vi "Get Camera Configuration.vi"(8 "error in (no error)":errorcluster, 11 "NI Vision Camera Device in":refnum<class "NI Vision Camera Device.lvclass">) -> (0 "error out":errorcluster, 2 "Configuration":T1, 3 "NI Vision Camera Device out":refnum<class "NI Vision Camera Device.lvclass">)   [LabVIEW 2014, in "NI Vision Camera Device.lvclass"]
uses:
  NI Vision Camera Device.lvclass
  Configuration.ctl
  NI Vision Camera Device.lvclass/NI Vision Camera Device.ctl
  <resource>/objmgr/imaqdx.rc
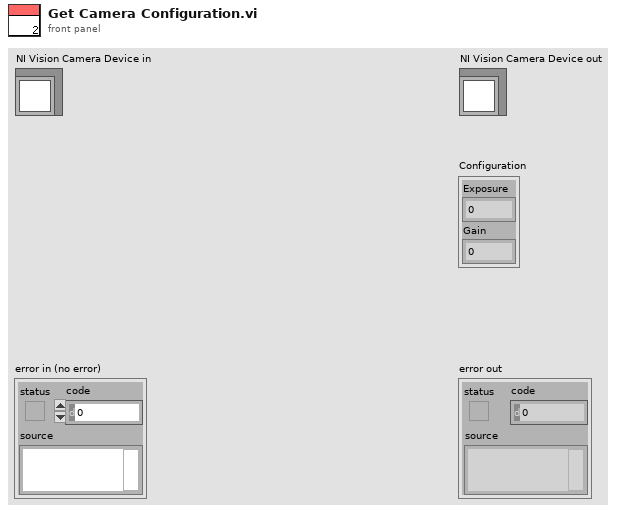
[diagram p1: front panel]
types:
  T1 = typedef "NI Vision Camera Device.lvclass/Configuration.ctl" = cluster{"Exposure":dbl, "Gain":dbl}
  T2 = typedef "IMAQdx.ctl" = refnum<k21>
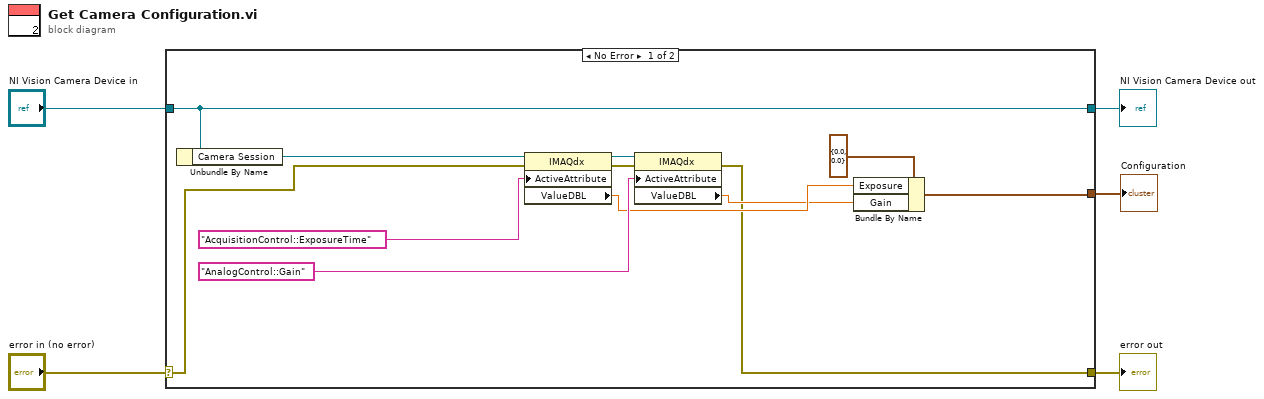
[diagram p0: block diagram]
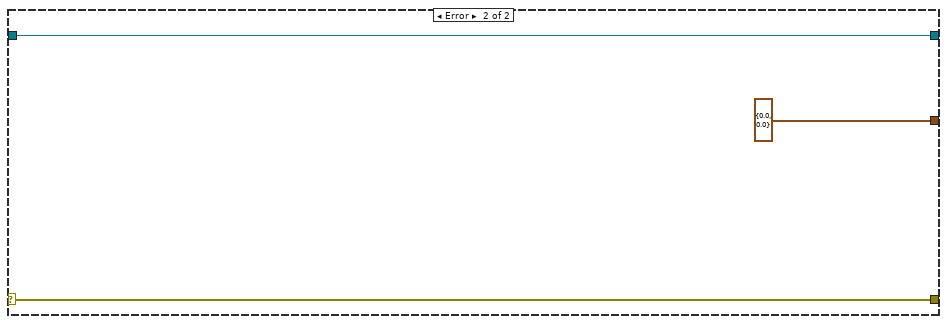
[diagram p2: hidden frame]
diagram:
  n1 = case shown="No Error" "error in (no error)" {
    selector: "error in (no error)" -> [w15 w20]
    tunnel: [w6 w20] -> w4
    tunnel: [w7 w19] -> w2
    tunnel: "NI Vision Camera Device in" -> [w7 w19]
    tunnel: [w9 T1 {"Exposure"=0.0, "Gain"=0.0} ("Configuration 2")] -> w1
    frame No Error {
      n2 = Unbundle By Name(w7) -> ("Camera Session"=w8:T2)
      n3 = property class="IMAQdx"(reference=w8, error in=w15, "ActiveAttribute"="AcquisitionControl::ExposureTime") -> (reference out=w17:T2, error out=w16:errorcluster, "ValueDBL"=w11:dbl)
      n4 = property class="IMAQdx"(reference=w17, error in=w16, "ActiveAttribute"="AnalogControl::Gain") -> (error out=w6:errorcluster, "ValueDBL"=w10:dbl)  [unwired: 1 out]
      n5 = Bundle By Name(cluster=T1 {"Exposure"=0.0, "Gain"=0.0} ("Configuration 2"), "Exposure"=w11, "Gain"=w10) -> (w9:T1)
    }
    frame Error {
    }
  }
  "error out" <- w4
  "NI Vision Camera Device out" <- w2
  "Configuration" <- w1
